vi "Sequence.CreateStopTask.vi"(8 "error in (no error)":errorcluster, 10 "Task Name":string, 11 "Task Ref":refnum<k24>) -> (0 "error out":errorcluster, 3 ".NET Refnum out":refnum<k24>)   [LabVIEW 2013, in "Simple Sequence Tools - Editor.lvlib"]
uses:
  Simple Sequence Tools - Editor.lvlib
  NationalInstruments.VeriStand.RealTimeSequenceDefinitionApi
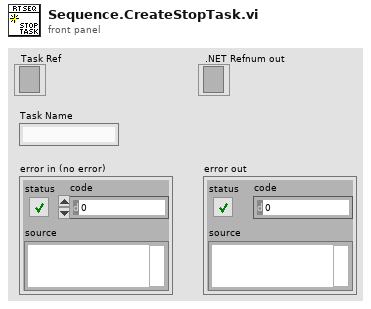
[diagram p1: front panel]
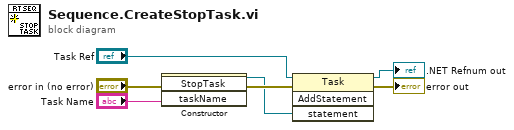
[diagram p0: block diagram]
diagram:
  n1 = constructor class="StopTask"(error in="error in (no error)", "taskName"="Task Name") -> (reference out=w4:refnum<k24>, error out=w6:errorcluster)  [unwired: 2 in, 2 out]
  n2 = invoke class="Task" method="AddStatement"(reference="Task Ref", error in=w6, "statement"=w4) -> (reference out=→".NET Refnum out":refnum<k24>, error out=→"error out":errorcluster)  [unwired: 1 in, 2 out]
